vi "getControlRef.vi"(8 "error in (no error)":errorcluster, 11 "Control in":refnum<class "Control.lvclass">) -> (0 "error out":errorcluster, 2 "controlRef":refnum<vi>, 3 "Control out":refnum<class "Control.lvclass">)   [LabVIEW 2023, in "TLC_Scripto.lvlib" / "Control.lvclass"]
uses:
  Control.lvclass
  Control.lvclass/Control.ctl
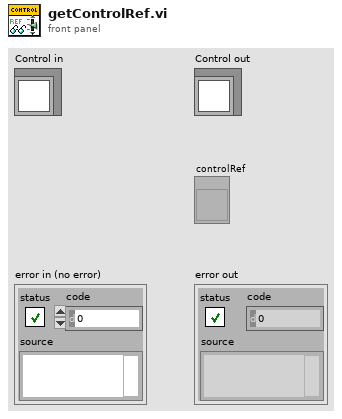
[diagram p1: front panel]
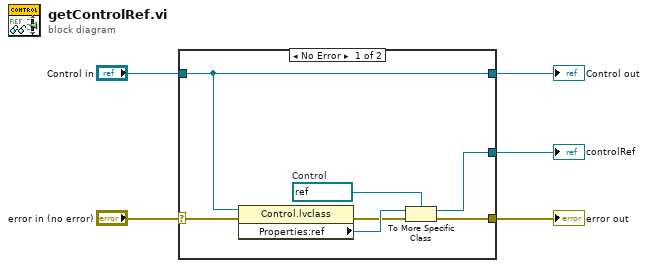
[diagram p0: block diagram]
diagram:
  n1 = case shown="No Error" "error in (no error)" {
    selector: "error in (no error)" -> [w7 w14]
    tunnel: [w10 w14] -> w4
    tunnel: [w12 w13] -> w2
    tunnel: "Control in" -> [w12 w13]
    tunnel: [w8 _] -> w1
    frame No Error {
      w9 = refnum<vi> refnum  # Control
      n2 = property class="Control.lvclass"(reference=w12, error in=w7) -> (error out=w6:errorcluster, "Properties:ref"=w11:refnum<vi>)  [unwired: 1 out]
      n3 = To More Specific Class(target class=w9, reference=w11, error in=w6) -> (specific class reference=w8:refnum<vi>, error out=w10:errorcluster)
    }
    frame Error {
    }
  }
  "error out" <- w4
  "Control out" <- w2
  "controlRef" <- w1
